vi "K to C and F demo.vi"() -> ()   [LabVIEW 2012]
panel:
  out "F":dbl[unit]=255.3722222222222
  out "C":dbl[unit]=273.15
  in  "K":dbl[unit]
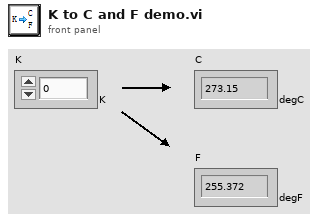
[diagram p1: front panel]
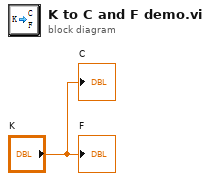
[diagram p0: block diagram]
diagram:
  "C" <- "K"
  "F" <- "K"
